vi "IND560 Serial Parse.vi"(8 "Error In":errorcluster, 11 "Weight Template":string="108.120 lb \r\n     0.000 lb T \r\n   108.120 lb N") -> (0 "Error Out":errorcluster, 2 "Net Weight":dbl, 3 "IND560 Serial Data":string[][](array[string]))   [LabVIEW 2023]
uses:
  <vilib>/Utility/error.llb/whitespace.ctl
  <vilib>/Utility/error.llb/Trim Whitespace One-Sided.vi
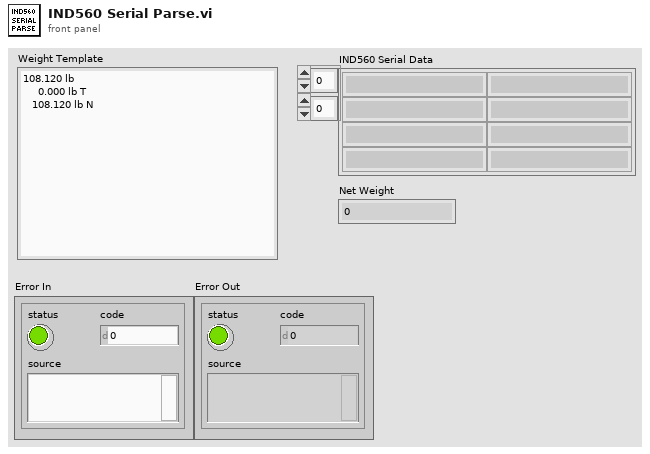
[diagram p1: front panel]
types:
  T1 = typedef "whitespace.ctl" = u16
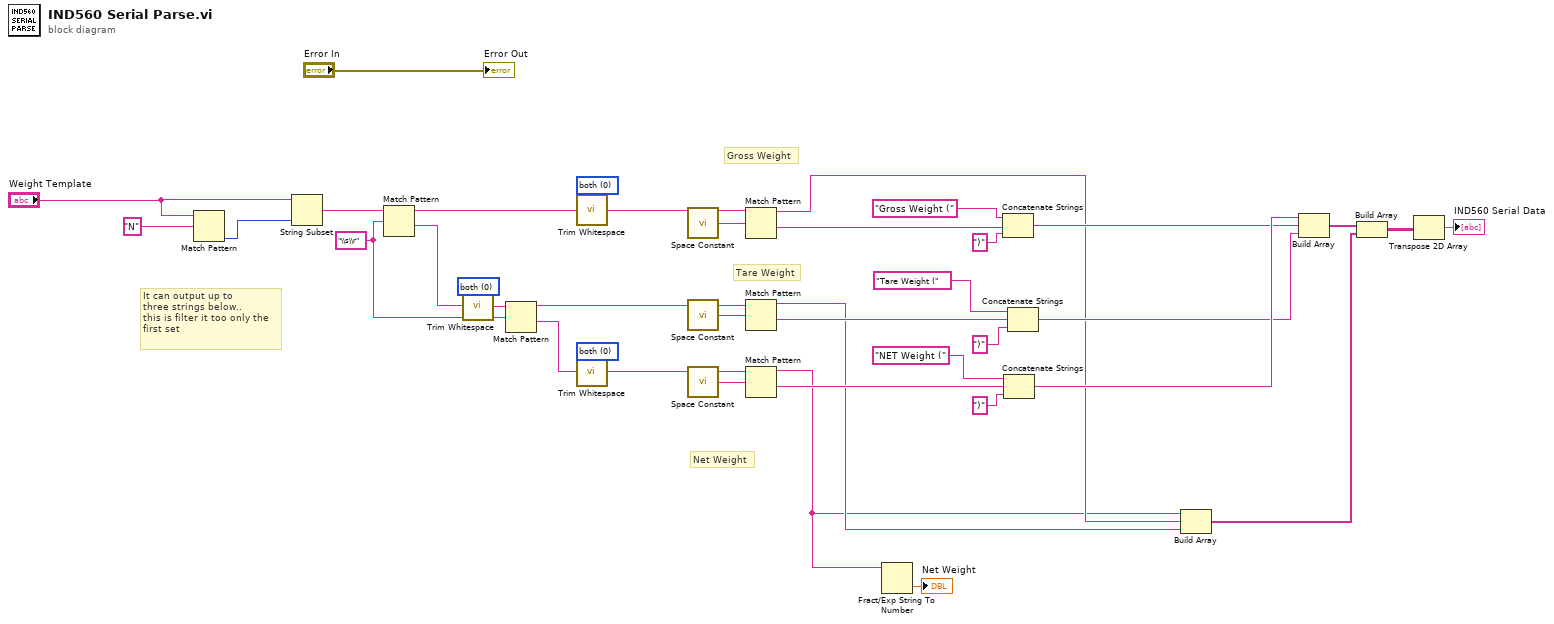
[diagram p0: block diagram]
diagram:
  w38 = T1 0 items=["both", "start of string", "end of string"] ("location (both)")
  w35 = T1 0 items=["both", "start of string", "end of string"] ("location (both)")
  w33 = T1 0 items=["both", "start of string", "end of string"] ("location (both)")
  w32 = "\\s\\r" ("regular expression")
  # "It can output up to \nthree strings below..\nthis is filter it too only the \nfirst set"
  # "Net Weight"
  # "Tare Weight"
  # "Gross Weight"
  n1 = Match Pattern(string="Weight Template", regular expression="N") -> (offset past match=w5:i32)  [unwired: 1 in, 3 out]
  n2 = String Subset(string="Weight Template", length (rest)=w5) -> (substring=w4:string)  [unwired: 1 in]
  n3 = Match Pattern(string=w4, regular expression=w32) -> (before substring=w34:string, after substring=w36:string)  [unwired: 1 in, 2 out]
  n4 = call <vilib>:"Trim Whitespace.vi"("string"=w36, "location (both)"=w35) -> ("trimmed string"=w37:string)
  n5 = Match Pattern(string=w37, regular expression=w32) -> (before substring=w27:string, after substring=w39:string)  [unwired: 1 in, 2 out]
  n6 = call <vilib>:"Trim Whitespace.vi"("string"=w34, "location (both)"=w33) -> ("trimmed string"=w30:string)
  n7 = call <vilib>:"Trim Whitespace.vi"("string"=w39, "location (both)"=w38) -> ("trimmed string"=w25:string)
  n8 = call <vilib>:"Space Constant.vi"() -> ("String"=w29:string)
  n9 = call <vilib>:"Space Constant.vi"() -> ("String"=w28:string)
  n10 = call <vilib>:"Space Constant.vi"() -> ("String"=w26:string)
  n11 = Match Pattern(string=w30, regular expression=w29) -> (before substring=w3:string, after substring=w12:string)  [unwired: 1 in, 2 out]
  n12 = Match Pattern(string=w27, regular expression=w28) -> (before substring=w11:string, after substring=w17:string)  [unwired: 1 in, 2 out]
  n13 = Match Pattern(string=w25, regular expression=w26) -> (before substring=w1:string, after substring=w23:string)  [unwired: 1 in, 2 out]
  n14 = Fract/Exp String To Number(string=w1) -> (number=→"Net Weight":dbl)  [unwired: 3 in, 1 out]
  n15 = Concatenate Strings("Gross Weight (" ("string"), w12, ")" ("string")) -> (w15:string)
  n16 = Concatenate Strings("NET Weight (" ("string"), w23, ")" ("string")) -> (w16:string)
  n17 = Concatenate Strings("Tare Weight (" ("string"), w17, ")" ("string")) -> (w14:string)
  n18 = Build Array(w1, w3, w11) -> (w10:string[])
  n19 = Build Array(w16, w15, w14) -> (w13:string[])
  n20 = Build Array(w13, w10) -> (w9:string[][])
  n21 = Transpose 2D Array(2D array=w9) -> (transposed array=→"IND560 Serial Data":string[][])
  "Error Out" <- "Error In"
